vi "Phase Calculator Initialization.vi"(6 "Feedback In":T1, 7 "Heel Strike?":bool, 8 "Hip Sum":dbl, 9 "Number of Samples":dbl, 10 "HS2":bool, 11 "HS1":bool) -> (4 "Feedback Out":T1)   [LabVIEW 2018]
uses:
  Phase Calculator Feedback Cluster.ctl
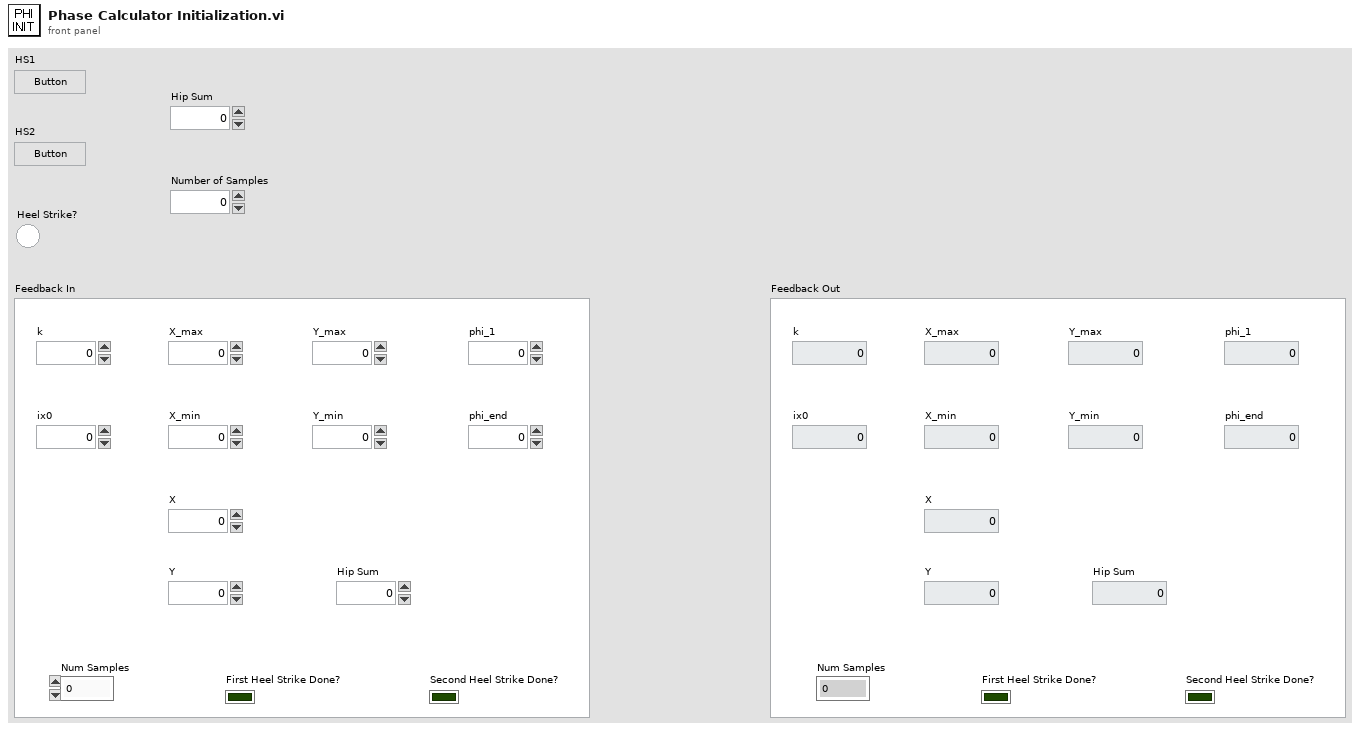
[diagram p1: front panel]
types:
  T1 = typedef "Phase Calculator Feedback Cluster.ctl" = cluster{"k":dbl, "ix0":dbl, "X_max":dbl, "X_min":dbl, "Y_max":dbl, "Y_min":dbl, "Y":dbl, "Hip Sum":dbl, "Num Samples":dbl, "First Heel Strike Done?":bool, "Second Heel Strike Done?":bool, "phi_1":dbl, "phi_end":dbl, "X":dbl}
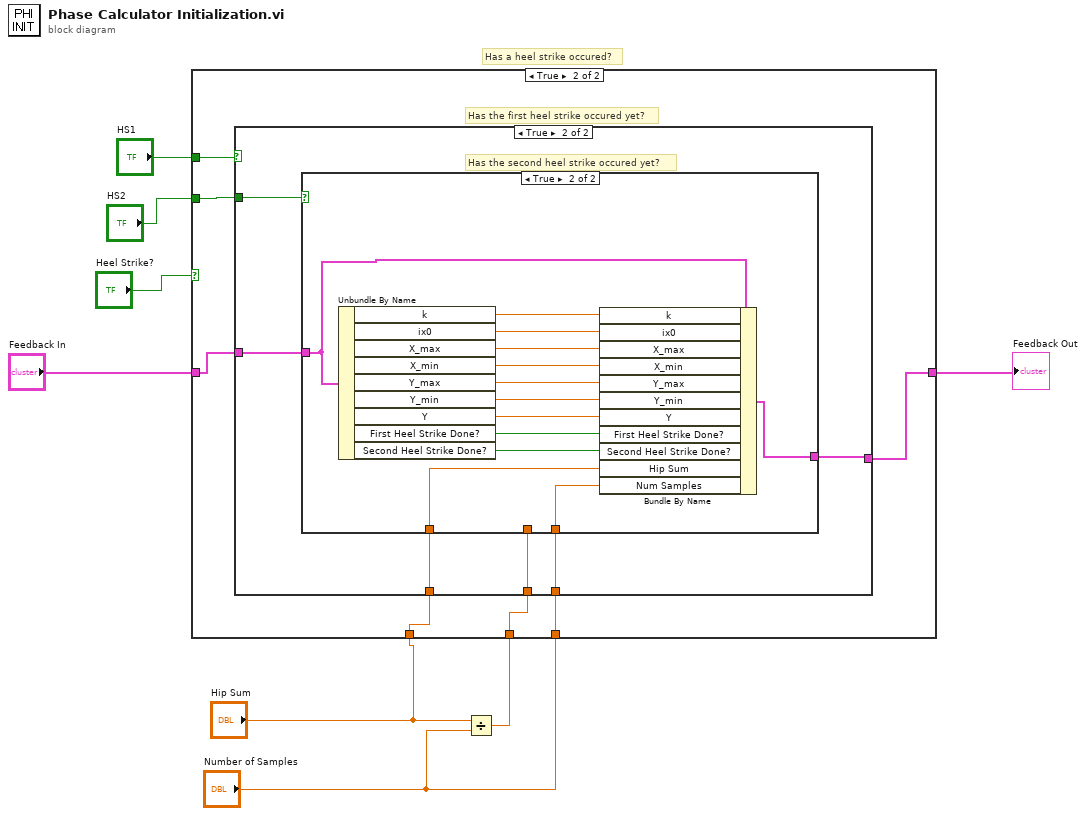
[diagram p0: block diagram]
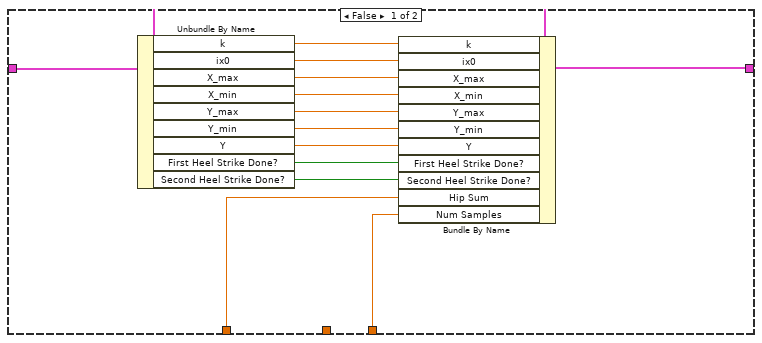
[diagram p2: hidden frame]
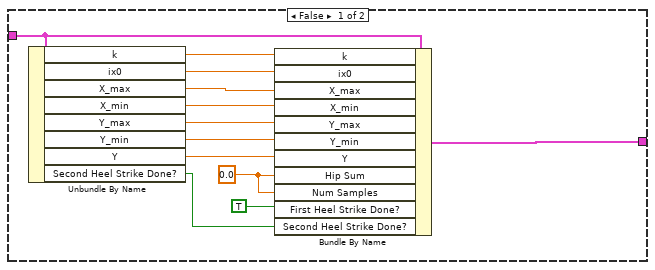
[diagram p3: hidden frame]
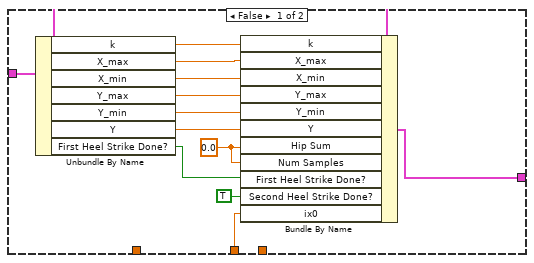
[diagram p4: hidden frame]
diagram:
  # "Has a heel strike occured?"
  n1 = Divide(x="Hip Sum", y="Number of Samples") -> (x/y=w3:dbl)
  n2 = case shown="True" "Heel Strike?" {
    tunnel: "HS1" -> [_ w28]
    tunnel: "HS2" -> [_ w27]
    tunnel: "Feedback In" -> [w20 w26]
    tunnel: [w21 w25] -> w4
    tunnel: w3 -> [_ w24]
    tunnel: "Hip Sum" -> [w10 w23]
    tunnel: "Number of Samples" -> [w9 w22]
    frame False {
      n3 = Unbundle By Name(w20) -> ("k"=w19:dbl, "ix0"=w18:dbl, "X_max"=w17:dbl, "X_min"=w16:dbl, "Y_max"=w15:dbl, "Y_min"=w14:dbl, "Y"=w13:dbl, "First Heel Strike Done?"=w12:bool, "Second Heel Strike Done?"=w11:bool)
      n4 = Bundle By Name(cluster=w20, "k"=w19, "ix0"=w18, "X_max"=w17, "X_min"=w16, "Y_max"=w15, "Y_min"=w14, "Y"=w13, "First Heel Strike Done?"=w12, "Second Heel Strike Done?"=w11, "Hip Sum"=w10, "Num Samples"=w9) -> (w21:T1)
    }
    frame True {
      # "Has the first heel strike occured yet?"
      n5 = case shown="True" w28 {
        tunnel: w27 -> [_ w46]
        tunnel: w26 -> [w39 w45]
        tunnel: [w30 w44] -> w25
        tunnel: w24 -> [_ w43]
        tunnel: w23 -> [_ w42]
        tunnel: w22 -> [_ w41]
        frame False {
          w31 = 0.0 ("Hip Sum")
          n6 = Unbundle By Name(w39) -> ("k"=w38:dbl, "ix0"=w37:dbl, "X_max"=w36:dbl, "X_min"=w35:dbl, "Y_max"=w34:dbl, "Y_min"=w33:dbl, "Y"=w32:dbl, "Second Heel Strike Done?"=w29:bool)
          n7 = Bundle By Name(cluster=w39, "k"=w38, "ix0"=w37, "X_max"=w36, "X_min"=w35, "Y_max"=w34, "Y_min"=w33, "Y"=w32, "Hip Sum"=w31, "Num Samples"=w31, "First Heel Strike Done?"=TRUE, "Second Heel Strike Done?"=w29) -> (w30:T1)
        }
        frame True {
          # "Has the second heel strike occured yet?"
          n8 = case shown="True" w46 {
            tunnel: w45 -> [w50 w59]
            tunnel: [w48 w62] -> w44
            tunnel: w43 -> [w49 _]
            tunnel: w42 -> [_ w61]
            tunnel: w41 -> [_ w60]
            frame False {
              w51 = 0.0 ("Hip Sum")
              n9 = Unbundle By Name(w50) -> ("k"=w57:dbl, "X_max"=w56:dbl, "X_min"=w55:dbl, "Y_max"=w54:dbl, "Y_min"=w53:dbl, "Y"=w52:dbl, "First Heel Strike Done?"=w47:bool)
              n10 = Bundle By Name(cluster=w50, "k"=w57, "X_max"=w56, "X_min"=w55, "Y_max"=w54, "Y_min"=w53, "Y"=w52, "Hip Sum"=w51, "Num Samples"=w51, "First Heel Strike Done?"=w47, "Second Heel Strike Done?"=TRUE, "ix0"=w49) -> (w48:T1)
            }
            frame True {
              n11 = Unbundle By Name(w59) -> ("k"=w71:dbl, "ix0"=w70:dbl, "X_max"=w69:dbl, "X_min"=w68:dbl, "Y_max"=w67:dbl, "Y_min"=w66:dbl, "Y"=w65:dbl, "First Heel Strike Done?"=w64:bool, "Second Heel Strike Done?"=w63:bool)
              n12 = Bundle By Name(cluster=w59, "k"=w71, "ix0"=w70, "X_max"=w69, "X_min"=w68, "Y_max"=w67, "Y_min"=w66, "Y"=w65, "First Heel Strike Done?"=w64, "Second Heel Strike Done?"=w63, "Hip Sum"=w61, "Num Samples"=w60) -> (w62:T1)
            }
          }
        }
      }
    }
  }
  "Feedback Out" <- w4
